vi "thermistorMain.vi"() -> ()   [LabVIEW 2023]
uses:
  <vilib>/Utility/file.llb/Write Delimited Spreadsheet (DBL).vi
  <vilib>/Analysis/NI_AALBase.lvlib
panel:
  out "temperature 2":dbl format="%0.2f"
  out "standard deviation":dbl format="%0.2f"
  out "mean":dbl format="%0.6e"
  in  "file path (dialog if empty)":path
  in  "stop":bool
  out "Temperature (deg C)":dbl(graph)
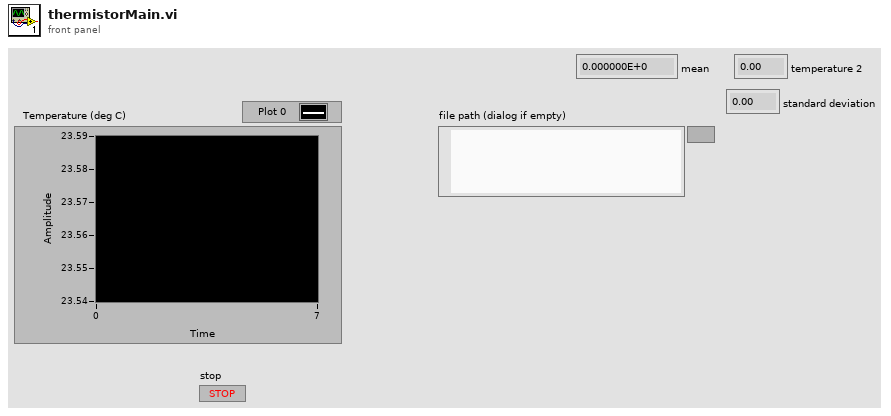
[diagram p1: front panel]
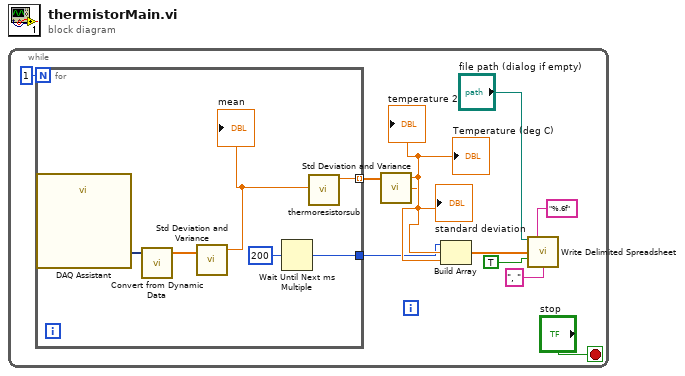
[diagram p0: block diagram]
diagram:
  n1 = while {
    stop <- "stop" stop-if-true
    n2 = for {
      N: 1 -> [_]
      tunnel: [w15] -> w6 mode=indexing
      tunnel: [w12] -> w1
      n3 = call "DAQ Assistant"() -> ("data"=w17:dynamicdata)  [unwired: 17 in, 2 out]
      n4 = call "Convert from Dynamic Data"("Dynamic Data Type"=w17) -> ("Array"=w16:dbl[])  [unwired: 3 in]
      n5 = call <vilib>:"Std Deviation and Variance.vi"("X"=w16) -> ("mean"=w14:dbl)  [unwired: 1 in, 2 out]
      "mean" <- w14
      n6 = Wait Until Next ms Multiple(millisecond multiple=u32 200) -> (millisecond timer value=w12:u32)
      n7 = call "thermoresistorsub.vi"("Input Voltage(mV)"=w14) -> ("output variable"=w15:dbl)  [unwired: 10 in]
    }
    n8 = call <vilib>:"Std Deviation and Variance.vi"("X"=w6) -> ("mean"=w5:dbl, "standard deviation"=w4:dbl)  [unwired: 1 in, 1 out]
    "Temperature (deg C)" <- w5
    "standard deviation" <- w4
    "temperature 2" <- w5
    n9 = Build Array(w1, w5, w4) -> (w10:dbl[])
    n10 = call-poly <vilib>:"Write Delimited Spreadsheet.vi"("file path (dialog if empty)"="file path (dialog if empty)", "format (%.3f)"="%.6f", "1D data"=w10, "append to file? (new file:F)"=TRUE, "delimiter (\\t)"=", " ("delimiter (\\t)")) -> ()  [unwired: 9 in, 2 out]
  }
